vi "Get Valid Test Num.vi"(8 "error in (no error)":errorcluster, 11 "Test Group in":refnum<class "Test Group.lvclass">) -> (0 "error out":errorcluster, 2 "Numeric":i32, 3 "Test Group out":refnum<class "Test Group.lvclass">)   [LabVIEW 2018, in "Test Number and Bin Generator.lvlib" / "Test Group.lvclass"]
uses:
  Test Group.lvclass
  Test Group.lvclass/Test Group.ctl
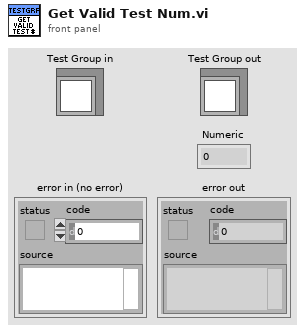
[diagram p1: front panel]
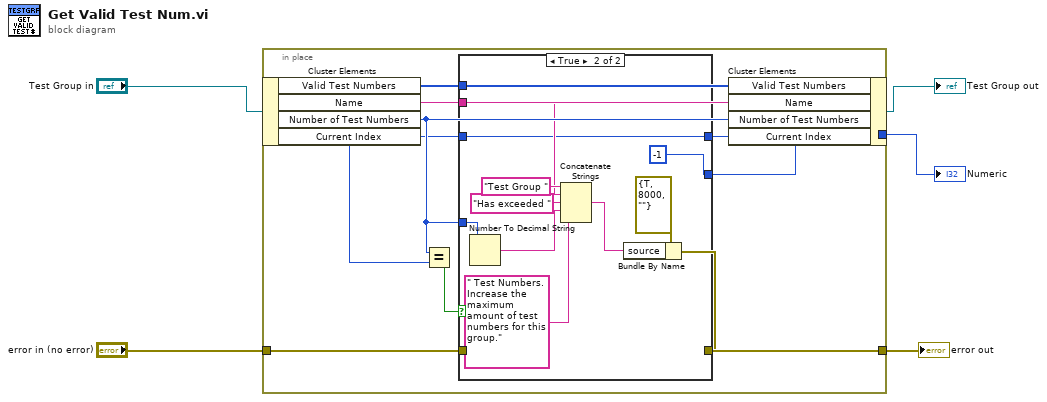
[diagram p0: block diagram]
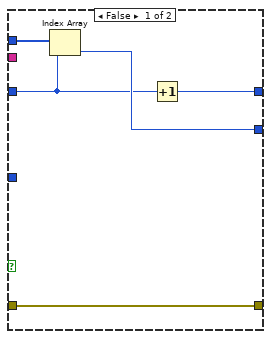
[diagram p2: hidden frame]
diagram:
  n1 = in-place {
    in-place-border: [w14] -> w1
    in-place-border: "error in (no error)" -> [w12]
    in-place-border: [w13] -> w4
    n2 = in-place-cluster #1("Test Group in") -> ("Valid Test Numbers"=w7:i32[], "Name"=w11:string, "Number of Test Numbers"=w10:i32, "Current Index"=w8:i32)
    n3 = Equal?(x=w10, y=w8) -> (x = y?=w9:bool)
    n4 = case shown="True" w9 {
      tunnel: [w19 -1 ("Numeric")] -> w14
      tunnel: w7 -> [w17 _]
      tunnel: [w18 w28] -> w13
      tunnel: w12 -> [w18 _]
      tunnel: w11 -> [_ w25]
      tunnel: w10 -> [_ w23]
      tunnel: w8 -> [w16 w20]
      tunnel: [w15 w20] -> w6
      frame False {
        n5 = Index Array(array=w17, index=w16) -> (element=w19:i32)
        n6 = Increment(x=w16) -> (x+1=w15:i32)
      }
      frame True {
        n7 = Number To Decimal String(number=w23) -> (decimal integer string=w22:string)  [unwired: 1 in]
        n8 = Concatenate Strings("Test Group " ("source"), w25, "Has exceeded " ("string"), w22, " Test Numbers.  Increase the maximum amount of test numbers for this group." ("string")) -> (w26:string)
        n9 = Bundle By Name(cluster=errorcluster {"status"=TRUE, "code"=8000, "source"=""} ("error IO"), "source"=w26) -> (w28:errorcluster)
      }
    }
    n10 = in-place-cluster #1("Valid Test Numbers"=w7, "Name"=w11, "Number of Test Numbers"=w10, "Current Index"=w6) -> (→"Test Group out":refnum<class "Test Group.lvclass">)
  }
  "error out" <- w4
  "Numeric" <- w1
